vi "GMLAN DeviceControl.vi"(8 "error in (no error)":errorcluster, 9 "CPIDControlBytes":u8[](array[numeric]) format="%.0x", 10 "CPID ID":u8 format="%.0x", 11 "diag ref in":T1={"Diag CAN Handle"=0, "Transport Protocol"=enum."ISO TP - Normal Mode", "Receive Address Extension"=0, "Transmit Address Extension"=0, "Receive CAN Id"=0, "Transmit CAN Id"=0, "Log Frames ?"=FALSE, "My TP Address"=0, "Other TP Address"=0, "T1"=0, "T2"=0, "T3"=0, "T4"=0, "Tx SN"=0, "Block Size"=0, "Rx SN"=0, "VW TP Initialized?"=FALSE, "Tx block no"=0, "baud rate"=0, "Interface"="", "Channel Diag CAN Handle"=0, "UDP Connection ID"=refnum, "TCP Connection ID"=refnum, "Target IP Addr"=0, "Source Address"=0, "Target Address"=0, "Send Header NACK?"=FALSE, "DLL Handle"=0, "NAD"=0, "Time Stamp read first"=0.0, "Time Stamp read last"=0.0, "Time Stamp write first"=0.0, "Time Stamp write last"=0.0, "Time Stamp write"=0.0, "Time Stamp read"=0.0, " I/O Mode"=0, "FD Baudrate"=0, "TX_DL"=8, "RX_DL"=8, "DoIP Protocol Version"=1, " Selected I/O Mode"=0, "TesterPresent Counter"=0, "TesterPresent Limit"=0, "TesterPresent Tick[ms]"=10, "TesterPresent RequireResponse?"=FALSE, "TesterPresent Stored Ref?"=FALSE, "TesterPresent Message"=[], "TesterPresent Task Handle"=0, "TesterPresent Semaphore"=refnum, "Response Plausibility Check"=1, "Default Version?"=TRUE, "Diagostic Globals"={"Timeout FC (Bs)"=250, "Timeout CF (Cr)"=250, "Timeout Diag Command"=1000, "Receive Block Size (BS)"=0, "Wait Time CF (STmin)"=5, "Max Waits (N_WFTmax)"=10, "Waits to Send (N_WAIT)"=0, "Time between Waits (TW)"=25, "Fill CAN Frames?"=TRUE, "Fill Byte"=255, "Invalid Response as Error?"=FALSE, "Max RspPending Count"=5, "VWTP Command Timeout"=50, "Transport Protocol"=enum."Diagnostics on IP", "Diag CAN Handle"=0, "DLL Handle"=0, "Timeout RspPending"=1000}, "Session-based Properties?"=FALSE} {"Diagostic Globals"."Fill Byte" format="%x"; "TesterPresent Message" format="%.0x"; "Selected I/O Mode" items=["CAN", "CAN FD", "CAN FD+BRS", "ECU Determined"]; "DoIP Protocol Version" items=["2010"=1, "2012"=2]; "RX_DL" items=["8"=8, "12"=12, "16"=16, "20"=20, "24"=24, "32"=32, "48"=48, "64"=64]; "TX_DL" items=["8"=8, "12"=12, "16"=16, "20"=20, "24"=24, "32"=32, "48"=48, "64"=64]; "I/O Mode" items=["CAN", "CAN FD", "CAN FD+BRS", "Not yet determined"]}) -> (0 "error out":errorcluster, 1 "success?":bool, 3 "diag ref out":T1={"Diag CAN Handle"=0, "Transport Protocol"=enum."ISO TP - Normal Mode", "Receive Address Extension"=0, "Transmit Address Extension"=0, "Receive CAN Id"=0, "Transmit CAN Id"=0, "Log Frames ?"=FALSE, "My TP Address"=0, "Other TP Address"=0, "T1"=0, "T2"=0, "T3"=0, "T4"=0, "Tx SN"=0, "Block Size"=0, "Rx SN"=0, "VW TP Initialized?"=FALSE, "Tx block no"=0, "baud rate"=0, "Interface"="", "Channel Diag CAN Handle"=0, "UDP Connection ID"=refnum, "TCP Connection ID"=refnum, "Target IP Addr"=0, "Source Address"=0, "Target Address"=0, "Send Header NACK?"=FALSE, "DLL Handle"=0, "NAD"=0, "Time Stamp read first"=0.0, "Time Stamp read last"=0.0, "Time Stamp write first"=0.0, "Time Stamp write last"=0.0, "Time Stamp write"=0.0, "Time Stamp read"=0.0, " I/O Mode"=0, "FD Baudrate"=0, "TX_DL"=8, "RX_DL"=8, "DoIP Protocol Version"=1, " Selected I/O Mode"=0, "TesterPresent Counter"=0, "TesterPresent Limit"=0, "TesterPresent Tick[ms]"=10, "TesterPresent RequireResponse?"=FALSE, "TesterPresent Stored Ref?"=FALSE, "TesterPresent Message"=[], "TesterPresent Task Handle"=0, "TesterPresent Semaphore"=refnum, "Response Plausibility Check"=1, "Default Version?"=TRUE, "Diagostic Globals"={"Timeout FC (Bs)"=250, "Timeout CF (Cr)"=250, "Timeout Diag Command"=1000, "Receive Block Size (BS)"=0, "Wait Time CF (STmin)"=5, "Max Waits (N_WFTmax)"=10, "Waits to Send (N_WAIT)"=0, "Time between Waits (TW)"=25, "Fill CAN Frames?"=TRUE, "Fill Byte"=255, "Invalid Response as Error?"=FALSE, "Max RspPending Count"=5, "VWTP Command Timeout"=50, "Transport Protocol"=enum."Diagnostics on IP", "Diag CAN Handle"=0, "DLL Handle"=0, "Timeout RspPending"=1000}, "Session-based Properties?"=FALSE} {"Diagostic Globals"."Fill Byte" format="%x"; "TesterPresent Message" format="%.0x"; "Selected I/O Mode" items=["CAN", "CAN FD", "CAN FD+BRS", "ECU Determined"]; "DoIP Protocol Version" items=["2010"=1, "2012"=2]; "RX_DL" items=["8"=8, "12"=12, "16"=16, "20"=20, "24"=24, "32"=32, "48"=48, "64"=64]; "TX_DL" items=["8"=8, "12"=12, "16"=16, "20"=20, "24"=24, "32"=32, "48"=48, "64"=64]; "I/O Mode" items=["CAN", "CAN FD", "CAN FD+BRS", "Not yet determined"]})   [LabVIEW 2019, in "GMLAN.lvlib"]
uses:
  GMLAN.lvlib
  <vilib>/Automotive Diagnostic Command Set/Diagnostic Transport.llb/Diag Reference.ctl
  <vilib>/Automotive Diagnostic Command Set/Diagnostic Transport.llb/Transport Protocol Selector.ctl
  <vilib>/Automotive Diagnostic Command Set/Diagnostic Transport.llb/DoIP Protocol Version.ctl
  <vilib>/Automotive Diagnostic Command Set/Diagnostic Transport.llb/Diag Globals.ctl
  <vilib>/addons/Automotive Diagnostic Command Set/NI_Automotive Diagnostic Command Set.lvlib
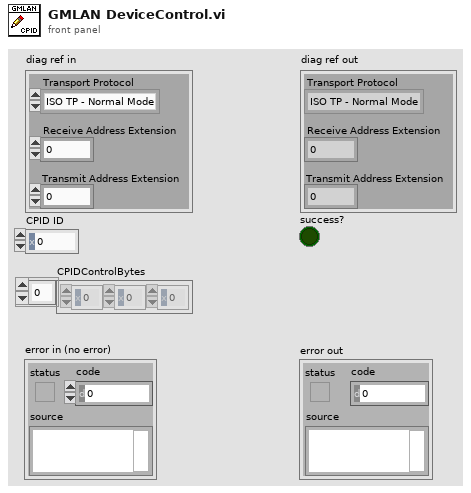
[diagram p1: front panel]
types:
  T1 = typedef "NI_Automotive Diagnostic Command Set.lvlib/Diag Reference.ctl" = cluster{"Diag CAN Handle":u32, "Transport Protocol":T2, "Receive Address Extension":u8, "Transmit Address Extension":u8, "Receive CAN Id":u32, "Transmit CAN Id":u32, "Log Frames ?":bool, "My TP Address":u8, "Other TP Address":u8, "T1":u16, "T2":u16, "T3":u16, "T4":u16, "Tx SN":u8, "Block Size":u8, "Rx SN":u8, "VW TP Initialized?":bool, "Tx block no":u8, "baud rate":u64, "Interface":string, "Channel Diag CAN Handle":u32, "UDP Connection ID":refnum<k16>, "TCP Connection ID":refnum<k5>, "Target IP Addr":u32, "Source Address":u16, "Target Address":u16, "Send Header NACK?":bool, "DLL Handle":u32, "NAD":u8, "Time Stamp read first":dbl, "Time Stamp read last":dbl, "Time Stamp write first":dbl, "Time Stamp write last":dbl, "Time Stamp write":dbl, "Time Stamp read":dbl, " I/O Mode":u32, "FD Baudrate":u64, "TX_DL":u16, "RX_DL":u16, "DoIP Protocol Version":T3, " Selected I/O Mode":u32, "TesterPresent Counter":u32, "TesterPresent Limit":u32, "TesterPresent Tick[ms]":i32, "TesterPresent RequireResponse?":bool, "TesterPresent Stored Ref?":bool, "TesterPresent Message":u8[], "TesterPresent Task Handle":i32, "TesterPresent Semaphore":T4, "Response Plausibility Check":u32, "Default Version?":bool, "Diagostic Globals":T5, "Session-based Properties?":bool}
  T2 = typedef "NI_Automotive Diagnostic Command Set.lvlib/Transport Protocol Selector.ctl" = enum16{"ISO TP - Normal Mode", "ISO TP - Mixed Mode", "VW TP 2.0", "Diagnostics on IP", "ISO TP LIN"}
  T3 = typedef "NI_Automotive Diagnostic Command Set.lvlib/DoIP Protocol Version.ctl" = u8
  T4 = typedef "Semaphore RefNum" = refnum<k1>
  T5 = typedef "NI_Automotive Diagnostic Command Set.lvlib/Diag Globals.ctl" = cluster{"Timeout FC (Bs)":u32, "Timeout CF (Cr)":u32, "Timeout Diag Command":u32, "Receive Block Size (BS)":u8, "Wait Time CF (STmin)":u8, "Max Waits (N_WFTmax)":u8, "Waits to Send (N_WAIT)":i32, "Time between Waits (TW)":u32, "Fill CAN Frames?":bool, "Fill Byte":u32, "Invalid Response as Error?":bool, "Max RspPending Count":u32, "VWTP Command Timeout":u32, "Transport Protocol":T2, "Diag CAN Handle":u32, "DLL Handle":u32, "Timeout RspPending":u32}
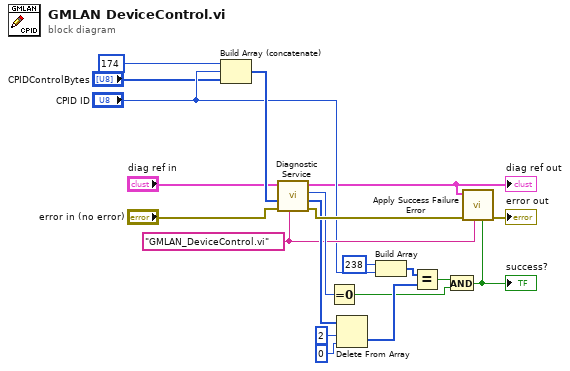
[diagram p0: block diagram]
diagram:
  w4 = "GMLAN_DeviceControl.vi" ("error source")
  n1 = Build Array (concatenate)(u8 174 ("element"), "CPID ID", "CPIDControlBytes") -> (w17:u8[])
  n2 = call <vilib>:"Diagnostic Service.vi"("error source"=w4, "error in (no error)"="error in (no error)", "data in"=w17, "diag ref in"="diag ref in") -> ("error out"=w19:errorcluster, "data out"=w11:u8[], "error code"=w16:u8, "diag ref out"=w1:T1)  [unwired: 2 in, 2 out]
  "diag ref out" <- w1
  n3 = Equal To 0?(x=w16) -> (x = 0?=w9:bool)
  n4 = Delete From Array(array=w11, length=2, index=0) -> (deleted portion=w10:u8[])  [unwired: 1 out]
  n5 = Build Array(u8 238 ("element"), "CPID ID") -> (w12:u8[])
  n6 = Equal?(x=w12, y=w10) -> (x = y?=w8:bool)
  n7 = And(x=w8, y=w9) -> (x .and. y?=w5:bool)
  "success?" <- w5
  n8 = call <vilib>:"Apply Success Failure Error.vi"("success code"=w5, "error source"=w4, "error in (no error)"=w19, "Diag Reference"=w1) -> ("error out"=→"error out":errorcluster)  [unwired: 7 out]
